vi "NPC3SG Labview V8.5.vi"(0 "dc level 1 in":refnum<vi>, 1 "dc level 2 in":refnum<vi>, 2 "dc level 3 in":refnum<vi>, 3 "loop 1 in":refnum<vi>, 4 "loop 2 in":refnum<vi>, 5 "loop 3 in":refnum<vi>, 6 "Port":refnum<visa-resource-name>="COM1", 7 "command in":refnum<vi>, 14 "dc level 1 out":refnum<vi>, 15 "dc level 2 out":refnum<vi>, 16 "dc level 3 out":refnum<vi>) -> ()   [LabVIEW 2015]
uses:
  SubNPC3SG.llb/device variables.vi
panel:
  in  "Stopp":bool
  in  "Registerkarte":T1(tab)
  in  "Loop 2":bool caption="Loop"
  in  "Remote 2":bool caption="Remote"
  in  "Loop 1":bool caption="Loop"
  in  "Remote 1":bool caption="Remote"
  in  "Remote 0":bool caption="Remote"
  in  "Loop 0":bool caption="Loop"
  in  "Refresh":bool
  out "Serial Number":string="RS232"
  out "Firmware Release Date":string="RS232"
  out "Version Number":string="RS232"
  out "Device":string="RS232"
  in  "com-write":bool caption="Logging"
  out "Receive Buffer":string
  out "Send Buffer":string
  in  "SendString":string caption="Enter Command"
  in  "Send":bool caption="Temp"
  in  "Clear":bool caption="Temp"
  out "Last Error":string="RS232"
  out "Last Command":string="RS232" caption="Command"
  in  "save sequence":bool caption="Loop"
  in  "load sequence":bool caption="Loop"
  in  "start sequence":bool caption="Loop"
  in  "sequence string":string
  in  "Drehschalter 2":dbl(knob) caption="2" min=-10.0 max=90.0 scale=0.0..100.0 scale format="%.3f"
  in  "Drehschalter 1":dbl(knob) caption="1" min=-10.0 max=90.0 scale=0.0..100.0 scale format="%.3f"
  in  "Drehschalter 0":dbl(knob) caption="0" min=-10.0 max=90.0 scale=0.0..100.0 scale format="%.3f"
  # "Piezo 1"
  # "Piezo 2"
  # "Piezo 3"
  # "Loop"
  # "Remote"
  # "possible commands in sequence\n\nset,1,2.34 (actuator position)\nwait,5  - (holding time in sec.)\nstop - (terminate sequence)\n\nexample:\nset,1,2.134\nwait,5\nset,0,22.66\nwait,10\nstop"
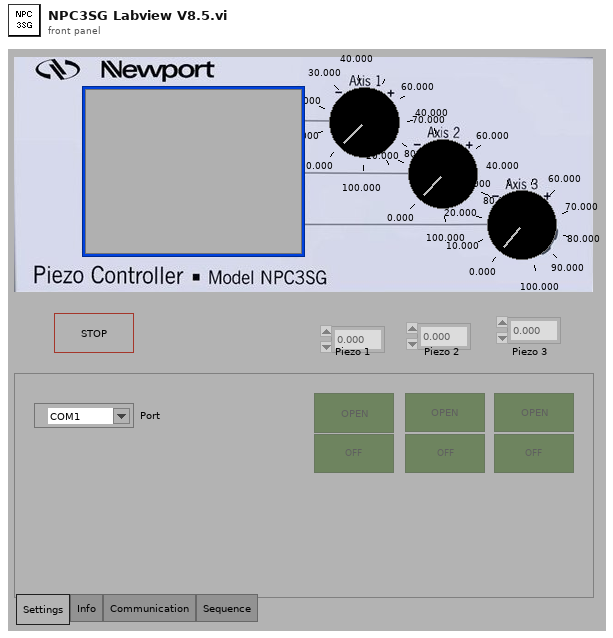
[diagram p1: front panel]
types:
  T1 = enum32{"Settings", "Info", "Communication", "Sequence"}
  T2 = enum16{"open", "replace", "create", "open or create", "replace or create", "replace or create with confirmation"}
  T3 = cluster{"Registerkarte":refnum<vi>, "Array IsActor":bool[], "Array loop":bool[], "Array remote":bool[]}
  T4 = cluster{"Array dc-level":dbl[], "VAR Temp":string, "VAR USB":string, "Array IsActor":bool[], "Array actor-name":string[], "Array axis":string[], "Array loop":bool[], "Array remote":bool[], "Array ovl":bool[]}
  T5 = cluster{"Drehschalter 0":refnum<vi>, "Drehschalter 1":refnum<vi>, "Drehschalter 2":refnum<vi>, "Array loop":bool[], "Array IsActor":bool[], "Array clmin":dbl[], "Array clmax":dbl[], "VAR Vmin":dbl, "VAR Vmax":dbl, "Array dc-level open":dbl[], "Array dc-level closed":dbl[], "VAR actualisation":bool}
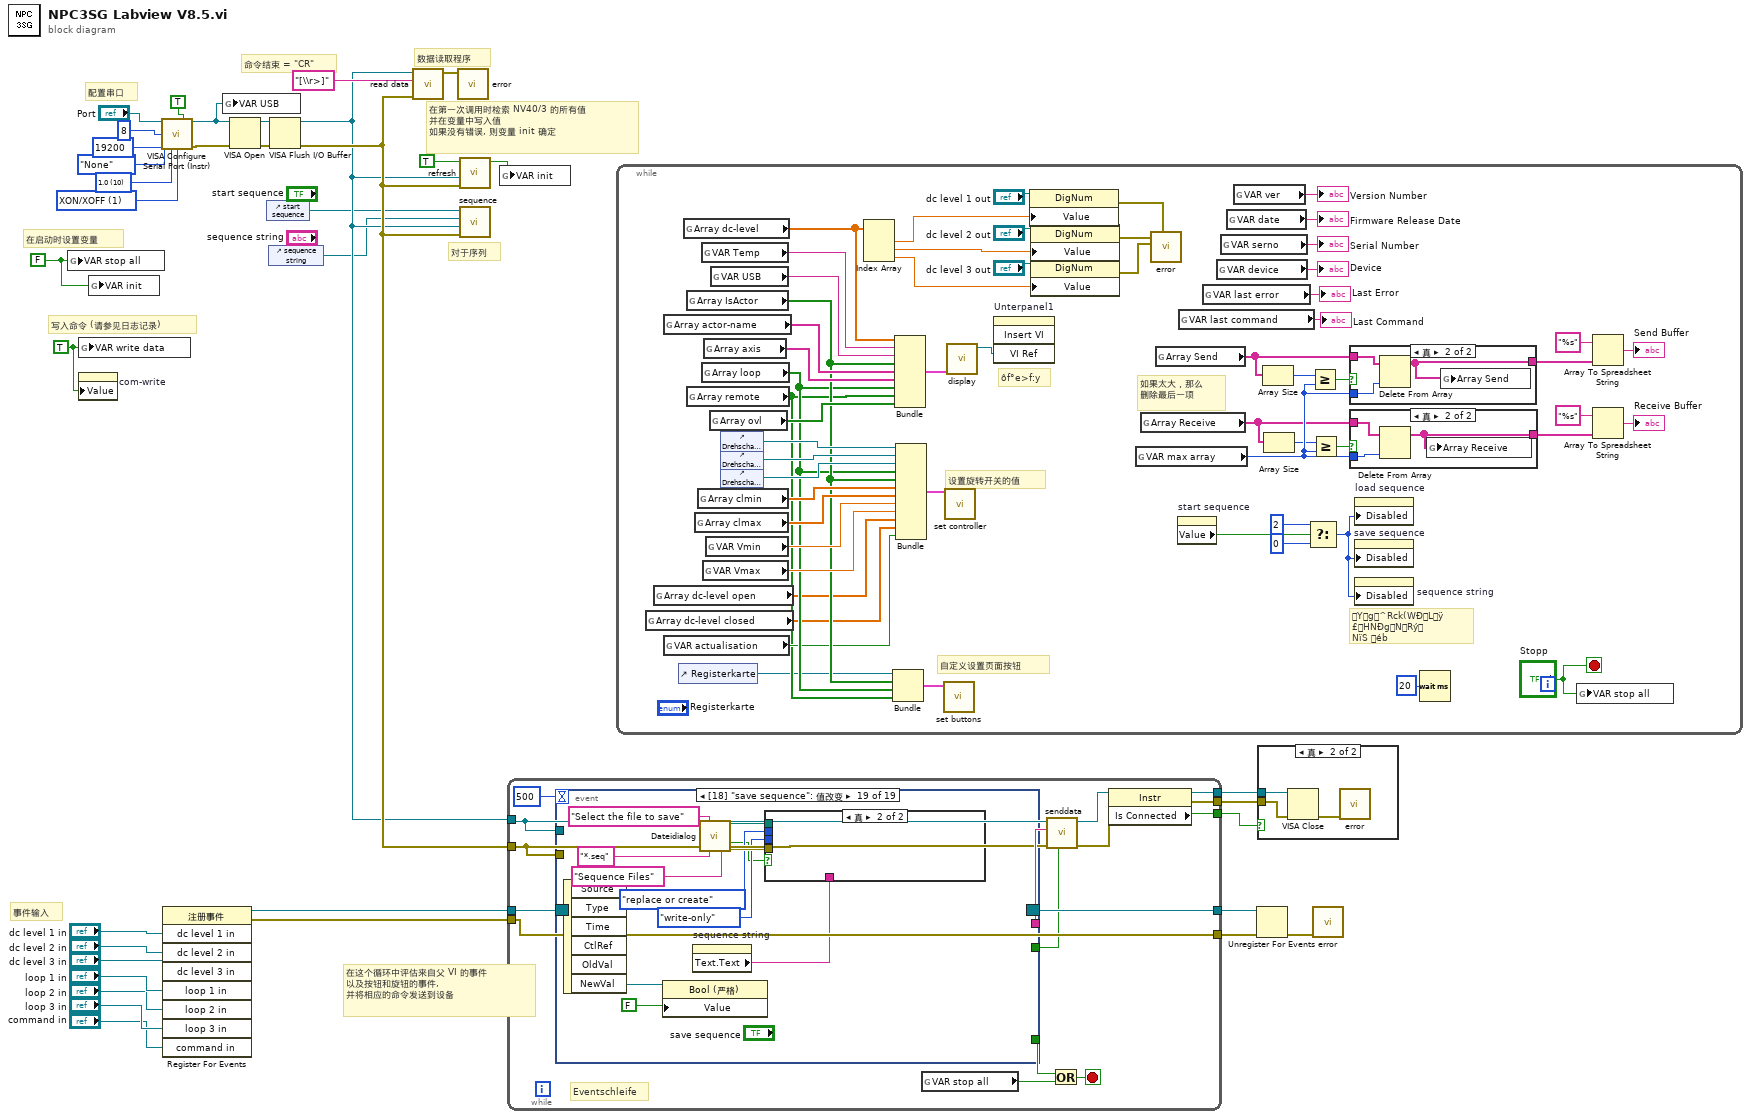
[diagram p0: block diagram]
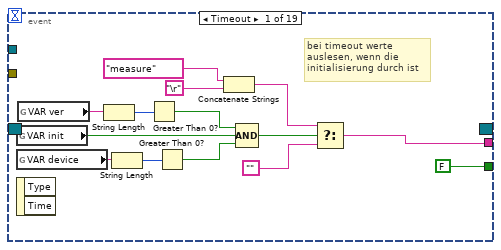
[diagram p3: hidden frame]
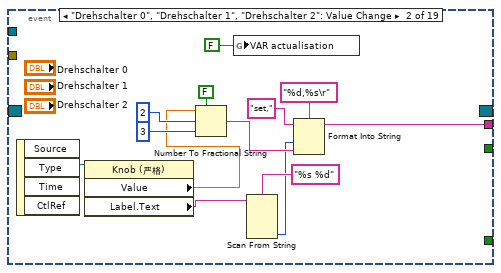
[diagram p4: hidden frame]
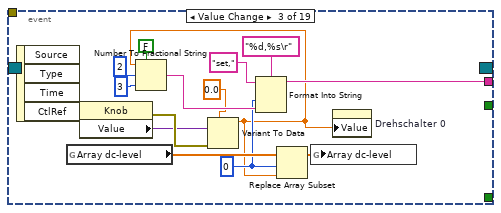
[diagram p5: hidden frame]
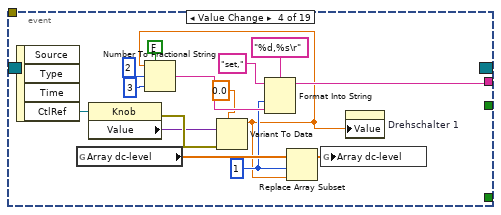
[diagram p6: hidden frame]
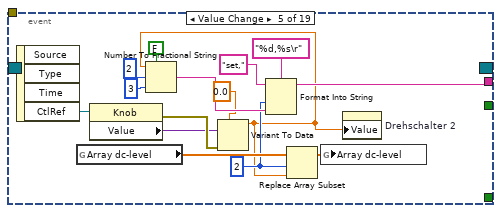
[diagram p7: hidden frame]
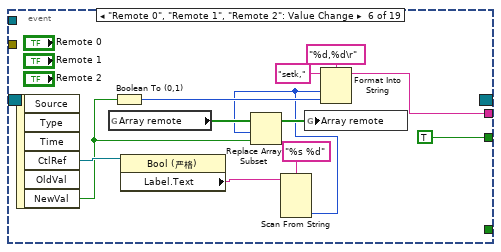
[diagram p8: hidden frame]
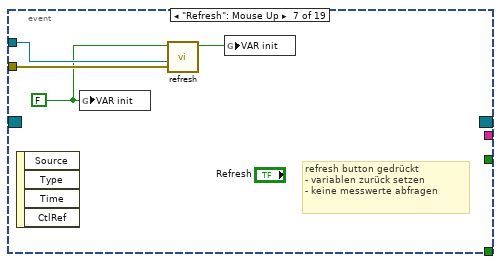
[diagram p9: hidden frame]
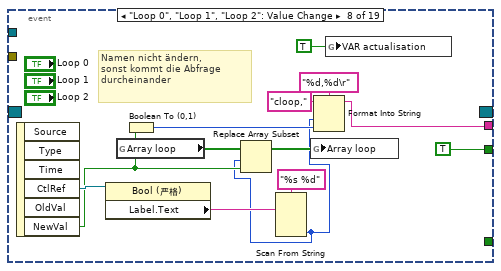
[diagram p10: hidden frame]
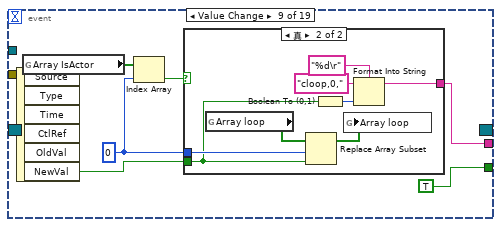
[diagram p11: hidden frame]
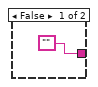
[diagram p12: hidden frame]
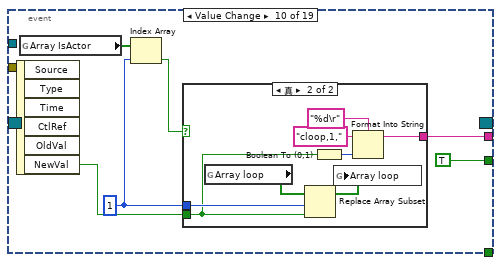
[diagram p13: hidden frame]
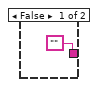
[diagram p14: hidden frame]
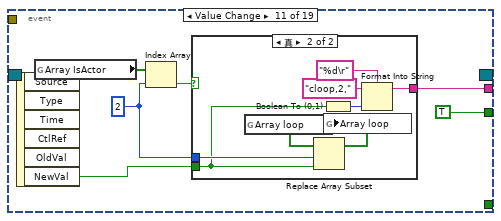
[diagram p15: hidden frame]
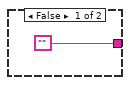
[diagram p16: hidden frame]
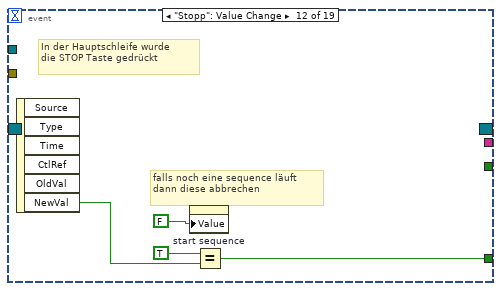
[diagram p17: hidden frame]
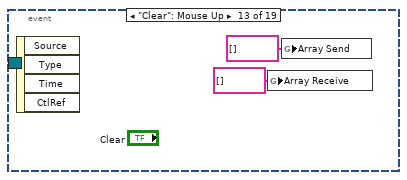
[diagram p18: hidden frame]
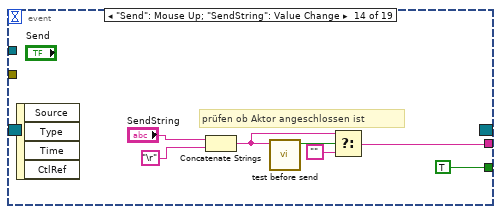
[diagram p19: hidden frame]
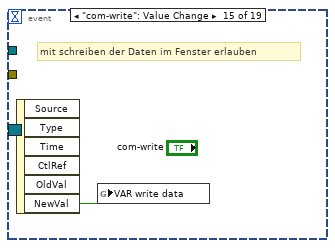
[diagram p20: hidden frame]
diagram:
  w9 = TRUE ("VAR write data")
  w13 = FALSE ("VAR ovl 3")
  w10 = u16 1 items=["Kein", "XON/XOFF", "RTS/CTS", "XON/XOFF & RTS/CTS", "DTR/DSR", "XON/XOFF & DTR/DSR"] ("flow control (0:none)")
  w29 = u16 10 items=["1.0"=10, "1.5"=15, "2.0"=20] ("stop bits (10: 1 bit)")
  # "对于序列"
  # "写入命令 (请参见日志记录)"
  # "命令结束 = \"CR\""
  # "数据读取程序"
  # "在第一次调用时检索 NV40/3 的所有值\n并在变量中写入值\n如果没有错误, 则变量 init 确定"
  # "在启动时设置变量"
  # "配置串口"
  # "事件输入"
  # "在这个循环中评估来自父 VI 的事件\n以及按钮和旋钮的事件, \n并将相应的命令发送到设备"
  n1 = global write "device variables.vi" "VAR stop all"(w13) -> ()
  n2 = global write "device variables.vi" "VAR write data"(w9) -> ()
  n3 = property on="com-write" class="Bool (严格)"("Value"=w9) -> ()  [unwired: 2 in, 2 out]
  n4 = global write "device variables.vi" "VAR init"(w13) -> ()
  n5 = call <vilib>:"VISA Configure Serial Port (Instr).vi"("VISA resource name"="Port", "Enable Termination\nChar (T)"=TRUE ("Enable Termination\nChar (T)"), "baud rate (9600)"=u32 19200, "data bits (8)"=u16 8, "parity (0:none)"=enum16{"None", "Odd", "Even", "Mark", "Space"}."None", "stop bits (10: 1 bit)"=w29, "flow control (0:none)"=w10) -> ("VISA resource name out"=w6:refnum<visa-resource-name>, "error out"=w18:errorcluster)  [unwired: 7 in]
  n6 = register-events("dc level 1 in", "dc level 2 in", "dc level 3 in", "loop 1 in", "loop 2 in", "loop 3 in", "command in") -> (reference out=w35:refnum<event-registration>, error out=w24:errorcluster)  [unwired: 2 in]
  n7 = global write "device variables.vi" "VAR USB"(w6) -> ()
  n8 = VISA Open(error in (no error)=w18, VISA resource name=w6) -> (VISA resource name=w19:refnum<visa-resource-name>, error out=w20:errorcluster)  [unwired: 3 in]
  n9 = control-ref of="start sequence"() -> (w2:refnum<vi>)
  n10 = control-ref of="sequence string"() -> (w1:refnum<vi>)
  n11 = VISA Flush I/O Buffer(VISA resource name=w19, error in (no error)=w20) -> (VISA resource name out=w3:refnum<visa-resource-name>, error out=w4:errorcluster)  [unwired: 1 in]
  n12 = call "read data.vi"("VISA resource name in"=w3, "String End"="[\\r>]", "error in"=w4) -> ("error ende"=w11:errorcluster)  [unwired: 7 in]
  n13 = call "error.vi"("error 1"=w11) -> ()  [unwired: 11 in]
  n14 = call "refresh.vi"("error in"=w4, "VISA-Ressourcen-Name (In)"=w3, "reset all"=TRUE) -> ("init ok??"=w8:bool)  [unwired: 8 in]
  n15 = call "sequence.vi"("error in"=w4, "VISA-Ressourcen-Name"=w3, "Kommandozeilen Refnum"=w1, "Startbutton Refnum"=w2) -> ()  [unwired: 8 in]
  n16 = global write "device variables.vi" "VAR init"(w8) -> ()
  n17 = while {
    tunnel: w4 -> [w38]
    tunnel: w3 -> [w39]
    tunnel: w35 -> [w47]
    tunnel: w24 -> [w40]
    tunnel: [w46] -> w23
    tunnel: [w40] -> w22
    tunnel: [w43] -> w16
    tunnel: [w42] -> w15
    tunnel: [w41] -> w14
    stop <- w49 stop-if-true
    # "Eventschleife"
    n18 = event shown="[18] \"save sequence\": 值改变" {
      selector: w47 -> [_ _ _ _ _ _ _ _ _ _ _ _ _ _ _ _ _ _ _]
      dyn-events: [_ _ _ _ _ _ _ _ _ _ _ _ _ _ _ _ _ _ _] -> w46
      timeout: 500 -> [_ _ _ _ _ _ _ _ _ _ _ _ _ _ _ _ _ _ _]
      tunnel: [w58 w74 w87 w99 w114 w129 _ w141 w157 w174 w188 _ _ w207 _ w214 _ _ _] -> w52
      tunnel: [_ _ _ _ _ _ _ _ _ _ _ w201 _ _ _ _ _ _ _] -> w51
      tunnel: w39 -> [_ _ _ _ _ _ w140 _ _ _ _ _ _ _ _ _ _ _ _]
      tunnel: w38 -> [_ _ _ _ _ _ w139 _ _ _ _ _ _ _ _ _ _ _ _]
      tunnel: [FALSE _ _ _ _ TRUE _ TRUE TRUE TRUE TRUE _ _ TRUE _ TRUE _ _ _] -> w37
      event Timeout {
        # "bei timeout werte auslesen, wenn die initialisierung durch ist"
        n19 = global read "device variables.vi" "VAR init"() -> (w64:bool)
        n20 = global read "device variables.vi" "VAR device"() -> (w62:string)
        n21 = event-data() -> ()  [unwired: 1 in, 2 out]
        n22 = global read "device variables.vi" "VAR ver"() -> (w66:string)
        n23 = String Length(string=w66) -> (length=w65:i32)
        n24 = String Length(string=w62) -> (length=w63:i32)
        n25 = Greater Than 0?(x=w65) -> (x > 0?=w60:bool)
        n26 = Greater Than 0?(x=w63) -> (x > 0?=w61:bool)
        n27 = Concatenate Strings("measure" ("String"), "\r") -> (w55:string)
        n28 = Compound Arithmetic op=AND(w60, w64, w61) -> (w59:bool)
        n29 = Select(t=w55, s=w59, f="") -> (s? t:f=w58:string)
      }
      event "Drehschalter 0", "Drehschalter 1", "Drehschalter 2": Value Change {
        n30 = event-data() -> ("CtlRef"=w73:refnum<vi>)  [unwired: 1 in, 3 out]
        n31 = property class="Knob (严格)"(reference=w73) -> ("Value"=w69:dbl, "Label.Text"=w72:string)  [unwired: 1 in, 2 out]
        n32 = Number To Fractional String(use system decimal point (T)=FALSE ("Systemdezimalzeichen verwenden (T)"), number=w69, width (-)=i16 2 ("Breite (-)"), precision (6)=i16 3 ("Genauigkeit (6)")) -> (F-format string=w70:string)
        n33 = global write "device variables.vi" "VAR actualisation"(FALSE ("VAR mode changed")) -> ()
        n34 = Scan From String(format string="%s %d" ("Format-String"), input string=w72) -> (output 2=w68:i32)  [unwired: 5 in, 3 out]
        n35 = Format Into String(format string="%d,%s\r", initial string="set,", w68, w70) -> (resulting string=w74:string)  [unwired: 1 in, 1 out]
      }
      event Value Change {
        w81 = u8 0 ("Eingang 1")
        n36 = event-data() -> ("CtlRef"=w94:refnum<vi>)  [unwired: 1 in, 3 out]
        n37 = global read "device variables.vi" "Array dc-level"() -> (w83:dbl[])
        n38 = property class="Knob"(reference=w94) -> (error out=w86:errorcluster, "Value"=w85:variant)  [unwired: 1 in, 1 out]
        n39 = Variant To Data(error in=w86, type=0.0, Variant=w85) -> (data=w80:dbl)  [unwired: 1 out]
        n40 = Number To Fractional String(use system decimal point (T)=FALSE ("Systemdezimalzeichen verwenden (T)"), number=w80, width (-)=i16 2 ("Breite (-)"), precision (6)=i16 3 ("Genauigkeit (6)")) -> (F-format string=w88:string)
        n41 = Format Into String(format string="%d,%s\r", initial string="set,", w81, w88) -> (resulting string=w87:string)  [unwired: 1 in, 1 out]
        n42 = Replace Array Subset(array=w83, new element=w80, index=w81) -> (w82:dbl[])
        n43 = global write "device variables.vi" "Array dc-level"(w82) -> ()
        n44 = property on="Drehschalter 0" class="Knob (严格)"("Value"=w80) -> ()  [unwired: 2 in, 2 out]
      }
      event Value Change {
        w96 = u8 1 ("Eingang 1")
        n45 = event-data() -> ("CtlRef"=w100:refnum<vi>)  [unwired: 1 in, 3 out]
        n46 = global read "device variables.vi" "Array dc-level"() -> (w98:dbl[])
        n47 = property class="Knob"(reference=w100) -> (error out=w103:errorcluster, "Value"=w102:variant)  [unwired: 1 in, 1 out]
        n48 = Variant To Data(error in=w103, type=0.0, Variant=w102) -> (data=w95:dbl)  [unwired: 1 out]
        n49 = Number To Fractional String(use system decimal point (T)=FALSE ("Systemdezimalzeichen verwenden (T)"), number=w95, width (-)=i16 2 ("Breite (-)"), precision (6)=i16 3 ("Genauigkeit (6)")) -> (F-format string=w104:string)
        n50 = Format Into String(format string="%d,%s\r", initial string="set,", w96, w104) -> (resulting string=w99:string)  [unwired: 1 in, 1 out]
        n51 = Replace Array Subset(array=w98, new element=w95, index=w96) -> (w97:dbl[])
        n52 = global write "device variables.vi" "Array dc-level"(w97) -> ()
        n53 = property on="Drehschalter 1" class="Knob (严格)"("Value"=w95) -> ()  [unwired: 2 in, 2 out]
      }
      event Value Change {
        w111 = u8 2 ("Eingang 1")
        n54 = event-data() -> ("CtlRef"=w115:refnum<vi>)  [unwired: 1 in, 3 out]
        n55 = global read "device variables.vi" "Array dc-level"() -> (w113:dbl[])
        n56 = property class="Knob"(reference=w115) -> (error out=w118:errorcluster, "Value"=w117:variant)  [unwired: 1 in, 1 out]
        n57 = Variant To Data(error in=w118, type=0.0, Variant=w117) -> (data=w110:dbl)  [unwired: 1 out]
        n58 = Number To Fractional String(use system decimal point (T)=FALSE ("Systemdezimalzeichen verwenden (T)"), number=w110, width (-)=i16 2 ("Breite (-)"), precision (6)=i16 3 ("Genauigkeit (6)")) -> (F-format string=w119:string)
        n59 = Format Into String(format string="%d,%s\r", initial string="set,", w111, w119) -> (resulting string=w114:string)  [unwired: 1 in, 1 out]
        n60 = Replace Array Subset(array=w113, new element=w110, index=w111) -> (w112:dbl[])
        n61 = global write "device variables.vi" "Array dc-level"(w112) -> ()
        n62 = property on="Drehschalter 2" class="Knob (严格)"("Value"=w110) -> ()  [unwired: 2 in, 2 out]
      }
      event "Remote 0", "Remote 1", "Remote 2": Value Change {
        n63 = event-data() -> ("CtlRef"=w134:refnum<vi>, "NewVal"=w126:bool)  [unwired: 1 in, 4 out]
        n64 = global read "device variables.vi" "Array remote"() -> (w135:bool[])
        n65 = Boolean To (0,1)(Boolean=w126) -> (0, 1=w130:i16)
        n66 = property class="Bool (严格)"(reference=w134) -> ("Label.Text"=w127:string)  [unwired: 1 in, 2 out]
        n67 = Scan From String(format string="%s %d" ("Format-String"), input string=w127) -> (output 2=w128:i32)  [unwired: 5 in, 3 out]
        n68 = Replace Array Subset(array=w135, new element=w126, index=w128) -> (w136:bool[])
        n69 = global write "device variables.vi" "Array remote"(w136) -> ()
        n70 = Format Into String(format string="%d,%d\r" ("Format-String"), initial string="setk,", w128, w130) -> (resulting string=w129:string)  [unwired: 1 in, 1 out]
      }
      event "Refresh": Mouse Up {
        w138 = FALSE ("VAR init")
        # "refresh button gedrückt\n- variablen zurück setzen\n- keine messwerte abfragen"
        n71 = event-data() -> ()  [unwired: 1 in, 4 out]
        n72 = global write "device variables.vi" "VAR init"(w138) -> ()
        n73 = call "refresh.vi"("error in"=w139, "VISA-Ressourcen-Name (In)"=w140, "reset all"=w138) -> ("init ok??"=w137:bool)  [unwired: 8 in]
        n74 = global write "device variables.vi" "VAR init"(w137) -> ()
      }
      event "Loop 0", "Loop 1", "Loop 2": Value Change {
        # "Namen nicht ändern,\nsonst kommt die Abfrage\ndurcheinander"
        n75 = event-data() -> ("CtlRef"=w147:refnum<vi>, "NewVal"=w146:bool)  [unwired: 1 in, 4 out]
        n76 = property class="Bool (严格)"(reference=w147) -> ("Label.Text"=w145:string)  [unwired: 1 in, 2 out]
        n77 = global read "device variables.vi" "Array loop"() -> (w152:bool[])
        n78 = Boolean To (0,1)(Boolean=w146) -> (0, 1=w148:i16)
        n79 = Scan From String(format string="%s %d" ("Format-String"), input string=w145) -> (output 2=w144:i32)  [unwired: 5 in, 3 out]
        n80 = Replace Array Subset(array=w152, new element=w146, index=w144) -> (w153:bool[])
        n81 = global write "device variables.vi" "Array loop"(w153) -> ()
        n82 = Format Into String(format string="%d,%d\r" ("Format-String"), initial string="cloop,", w144, w148) -> (resulting string=w141:string)  [unwired: 1 in, 1 out]
        n83 = global write "device variables.vi" "VAR actualisation"(TRUE ("VAR mode changed")) -> ()
      }
      event Value Change {
        w155 = 0 ("Index")
        n84 = event-data() -> ("NewVal"=w156:bool)  [unwired: 1 in, 5 out]
        n85 = global read "device variables.vi" "Array IsActor"() -> (w159:bool[])
        n86 = Index Array(array=w159, index=w155) -> (element=w158:bool)
        n87 = case shown="真" w158 {
          tunnel: ["" w166] -> w157
          tunnel: w156 -> [_ w161]
          tunnel: w155 -> [_ w163]
          frame False {
          }
          frame True {
            n88 = global read "device variables.vi" "Array loop"() -> (w165:bool[])
            n89 = Replace Array Subset(array=w165, new element=w161, index=w163) -> (w164:bool[])
            n90 = Boolean To (0,1)(Boolean=w161) -> (0, 1=w162:i16)
            n91 = global write "device variables.vi" "Array loop"(w164) -> ()
            n92 = Format Into String(format string="%d\r" ("Format-String"), initial string="cloop,0," ("Anfangsstring"), w162) -> (resulting string=w166:string)  [unwired: 1 in, 1 out]
          }
        }
      }
      event Value Change {
        w170 = 1
        n93 = event-data() -> ("NewVal"=w171:bool)  [unwired: 1 in, 5 out]
        n94 = global read "device variables.vi" "Array IsActor"() -> (w173:bool[])
        n95 = Index Array(array=w173, index=w170) -> (element=w172:bool)
        n96 = case shown="真" w172 {
          tunnel: ["" w181] -> w174
          tunnel: w171 -> [_ w176]
          tunnel: w170 -> [_ w178]
          frame False {
          }
          frame True {
            n97 = global read "device variables.vi" "Array loop"() -> (w180:bool[])
            n98 = Replace Array Subset(array=w180, new element=w176, index=w178) -> (w179:bool[])
            n99 = Boolean To (0,1)(Boolean=w176) -> (0, 1=w177:i16)
            n100 = global write "device variables.vi" "Array loop"(w179) -> ()
            n101 = Format Into String(format string="%d\r" ("Format-String"), initial string="cloop,1," ("Anfangsstring"), w177) -> (resulting string=w181:string)  [unwired: 1 in, 1 out]
          }
        }
      }
      event Value Change {
        w185 = 2
        n102 = event-data() -> ("NewVal"=w186:bool)  [unwired: 1 in, 5 out]
        n103 = global read "device variables.vi" "Array IsActor"() -> (w189:bool[])
        n104 = Index Array(array=w189, index=w185) -> (element=w187:bool)
        n105 = case shown="真" w187 {
          tunnel: ["" w196] -> w188
          tunnel: w186 -> [_ w191]
          tunnel: w185 -> [_ w193]
          frame False {
          }
          frame True {
            n106 = global read "device variables.vi" "Array loop"() -> (w195:bool[])
            n107 = Replace Array Subset(array=w195, new element=w191, index=w193) -> (w194:bool[])
            n108 = Boolean To (0,1)(Boolean=w191) -> (0, 1=w192:i16)
            n109 = global write "device variables.vi" "Array loop"(w194) -> ()
            n110 = Format Into String(format string="%d\r" ("Format-String"), initial string="cloop,2," ("Anfangsstring"), w192) -> (resulting string=w196:string)  [unwired: 1 in, 1 out]
          }
        }
      }
      event "Stopp": Value Change {
        # "falls noch eine sequence läuft\ndann diese abbrechen"
        # "In der Hauptschleife wurde\ndie STOP Taste gedrückt"
        n111 = event-data() -> ("NewVal"=w202:bool)  [unwired: 1 in, 5 out]
        n112 = property on="start sequence" class="Bool (严格)"("Value"=FALSE ("start sequence")) -> ()  [unwired: 2 in, 2 out]
        n113 = Equal?(x=TRUE, y=w202) -> (x = y?=w201:bool)
      }
      event "Clear": Mouse Up {
        n114 = event-data() -> ()  [unwired: 1 in, 4 out]
        n115 = global write "device variables.vi" "Array Receive"(string[] [] ("Array Receive")) -> ()
        n116 = global write "device variables.vi" "Array Send"(string[] [] ("Array Send")) -> ()
      }
      event "Send": Mouse Up; "SendString": Value Change {
        # "prüfen ob Aktor angeschlossen ist"
        n117 = event-data() -> ()  [unwired: 1 in, 4 out]
        n118 = Concatenate Strings("SendString", "\r") -> (w208:string)
        n119 = call "test before send.vi"("data string in"=w208) -> ("send OK"=w209:bool)  [unwired: 10 in]
        n120 = Select(t=w208, s=w209, f="") -> (s? t:f=w207:string)
      }
      event "com-write": Value Change {
        # "mit schreiben der Daten im Fenster erlauben"
        n121 = event-data() -> ("NewVal"=w212:bool)  [unwired: 1 in, 5 out]
        n122 = global write "device variables.vi" "VAR write data"(w212) -> ()
      }
      event Value Change {
        # "prüfen, ob Aktor angeschlossen"
        # "Kommando wurde von aussen geschickt"
        n123 = event-data() -> ("NewVal"=w219:string)  [unwired: 1 in, 5 out]
        n124 = Concatenate Strings(w219, "\r") -> (w216:string)
        n125 = call "test before send.vi"("data string in"=w216) -> ("send OK"=w217:bool)  [unwired: 10 in]
        n126 = Select(t=w216, s=w217, f="") -> (s? t:f=w214:string)
      }
      event "start sequence": Value Change {
        n127 = event-data() -> ()  [unwired: 1 in, 6 out]
      }
      event "load sequence": Value Change {
        n128 = event-data() -> ("CtlRef"=w221:refnum<vi>)  [unwired: 1 in, 5 out]
        n129 = property class="Bool (严格)"(reference=w221, "Value"=FALSE ("Wert")) -> ()  [unwired: 1 in, 2 out]
        n130 = call "Dateidialog2"("prompt"="Select the file to load", "pattern (all files)"="*.seq", "pattern label"="Sequence Files") -> ("selected path"=w227:path, "exists"=w223:bool, "error out"=w226:errorcluster)  [unwired: 9 in, 1 out]
        n131 = case shown="真" w223 {
          tunnel: w227 -> [_ w241]
          tunnel: w226 -> [_ w240]
          tunnel: T2."open" ("Operation (0:Öffnen)") -> [_ w238]
          tunnel: enum16{"read/write", "read-only", "write-only"}."read-only" ("Zugriff (0:Lesen/Schreiben)") -> [_ w237]
          tunnel: [w231 w232] -> w222
          frame False {
            (unwired) ""
            n132 = property on="sequence string" class="Str"() -> ("Text.Text"=w231:string)  [unwired: 2 in, 2 out]
          }
          frame True {
            n133 = Open/Create/Replace File(file path (use dialog)=w241, error in=w240, operation (0:open)=w238, access (0:read/write)=w237) -> (refnum out=w234:refnum<file>, error out=w233:errorcluster)  [unwired: 2 in, 1 out]
            n134 = Read from Text File(file (use dialog)=w234, error in=w233) -> (refnum out=w235:refnum<file>, text=w232:string, error out=w236:errorcluster)  [unwired: 2 in, 1 out]
            n135 = Close File(refnum=w235, error in=w236) -> (error out=w239:errorcluster)  [unwired: 1 out]
            n136 = call <vilib>:"Simple Error Handler.vi"("error in (no error)"=w239) -> ()  [unwired: 4 in, 5 out]
          }
        }
        n137 = property on="sequence string" class="Str"("Text.Text"=w222) -> ()  [unwired: 2 in, 2 out]
      }
      event "save sequence": Value Change {
        n138 = event-data() -> ("CtlRef"=w244:refnum<vi>)  [unwired: 1 in, 5 out]
        n139 = property class="Bool (严格)"(reference=w244, "Value"=FALSE ("Wert")) -> ()  [unwired: 1 in, 2 out]
        n140 = property on="sequence string" class="Str"() -> ("Text.Text"=w247:string)  [unwired: 2 in, 2 out]
        n141 = call "Dateidialog"("prompt"="Select the file to save", "pattern (all files)"="*.seq", "pattern label"="Sequence Files") -> ("selected path"=w249:path, "cancelled"=w242:bool, "error out"=w248:errorcluster)  [unwired: 9 in, 1 out]
        n142 = case shown="真" w242 {
          tunnel: w249 -> [w262 _]
          tunnel: w248 -> [w261 _]
          tunnel: w247 -> [w260 _]
          tunnel: T2."replace or create" ("Operation (0:Öffnen)") -> [w259 _]
          tunnel: enum16{"read/write", "read-only", "write-only"}."write-only" ("Zugriff (0:Lesen/Schreiben)") -> [w258 _]
          frame False {
            n143 = Open/Create/Replace File(file path (use dialog)=w262, error in=w261, operation (0:open)=w259, access (0:read/write)=w258) -> (refnum out=w257:refnum<file>, error out=w254:errorcluster)  [unwired: 2 in, 1 out]
            n144 = Write to Text File(file (use dialog)=w257, text=w260, error in=w254) -> (refnum out=w255:refnum<file>, error out=w256:errorcluster)  [unwired: 1 in, 1 out]
            n145 = Close File(refnum=w255, error in=w256) -> (error out=w253:errorcluster)  [unwired: 1 out]
            n146 = call <vilib>:"Simple Error Handler.vi"("error in (no error)"=w253) -> ()  [unwired: 4 in, 5 out]
          }
          frame True {
          }
        }
      }
    }
    n147 = global read "device variables.vi" "VAR stop all"() -> (w50:bool)
    n148 = call "senddata.vi"("read ERR"=w37, "error in"=w38, "writebuffer"=w52, "VISA-Ressourcen-Name"=w39) -> ("error out"=w44:errorcluster, "VISA-Ressourcen-Name (Ausgang)"=w45:refnum<visa-resource-name>)  [unwired: 5 in, 1 out]
    n149 = Or(x=w51, y=w50) -> (x .or. y?=w49:bool)
    n150 = property class="Instr"(reference=w45, error in=w44) -> (reference out=w43:refnum<visa-resource-name>, error out=w42:errorcluster, "Is Connected"=w41:bool)
  }
  n151 = while {
    stop <- "Stopp" stop-if-true
    # "Yg^Rck(WÐLÿ\n£HNÐgNRý\nNïS\téb"
    # "如果太大，那么\n删除最后一项"
    # "ôf°e>f:y"
    # "自定义设置页面按钮"
    # "设置旋转开关的值"
    n152 = global read "device variables.vi" "Array dc-level closed"() -> (w274:dbl[])
    n153 = global read "device variables.vi" "Array dc-level open"() -> (w275:dbl[])
    n154 = global read "device variables.vi" "Array actor-name"() -> (w316:string[])
    n155 = global read "device variables.vi" "VAR actualisation"() -> (w272:bool)
    n156 = control-ref of="Registerkarte"() -> (w270:refnum<vi>)
    n157 = global read "device variables.vi" "Array dc-level"() -> (w313:dbl[])
    n158 = global read "device variables.vi" "Array IsActor"() -> (w294:bool[])
    n159 = global read "device variables.vi" "Array remote"() -> (w271:bool[])
    n160 = global read "device variables.vi" "Array clmax"() -> (w301:dbl[])
    n161 = global read "device variables.vi" "Array clmin"() -> (w302:dbl[])
    n162 = global read "device variables.vi" "VAR Temp"() -> (w318:string)
    n163 = global read "device variables.vi" "Array loop"() -> (w293:bool[])
    n164 = global read "device variables.vi" "VAR Vmax"() -> (w299:dbl)
    n165 = global read "device variables.vi" "Array axis"() -> (w315:string[])
    n166 = global read "device variables.vi" "VAR Vmin"() -> (w300:dbl)
    n167 = global read "device variables.vi" "Array ovl"() -> (w314:bool[])
    n168 = global read "device variables.vi" "VAR USB"() -> (w317:string)
    n169 = control-ref of="Drehschalter 0"() -> (w298:refnum<vi>)
    n170 = control-ref of="Drehschalter 1"() -> (w297:refnum<vi>)
    n171 = control-ref of="Drehschalter 2"() -> (w296:refnum<vi>)
    n172 = Index Array(array=w313) -> (element #1=w312:dbl, element #2=w311:dbl, element #3=w310:dbl)  [unwired: 3 in]
    n173 = Bundle("Registerkarte"=w270, "Array IsActor"=w294, "Array loop"=w293, "Array remote"=w271) -> (w269:T3)  [unwired: 1 in]
    n174 = Bundle("Array dc-level"=w313, "VAR Temp"=w318, "VAR USB"=w317, "Array IsActor"=w294, "Array actor-name"=w316, "Array axis"=w315, "Array loop"=w293, "Array remote"=w271, "Array ovl"=w314) -> (w295:T4)  [unwired: 1 in]
    n175 = Bundle("Drehschalter 0"=w298, "Drehschalter 1"=w297, "Drehschalter 2"=w296, "Array loop"=w293, "Array IsActor"=w294, "Array clmin"=w302, "Array clmax"=w301, "VAR Vmin"=w300, "VAR Vmax"=w299, "Array dc-level open"=w275, "Array dc-level closed"=w274, "VAR actualisation"=w272) -> (w273:T5)  [unwired: 1 in]
    n176 = call "set buttons.vi"("Cluster Button"=w269) -> ()  [unwired: 11 in]
    n177 = call "set controller.vi"("Cluster Controller"=w273) -> ()  [unwired: 12 in, 3 out]
    n178 = call "display.vi"("Cluster Display In"=w295) -> ("Display - Refnum"=w319:refnum<vi>)  [unwired: 10 in]
    n179 = invoke on="Unterpanel1" class="SubPanel" method="Insert VI"("VI Ref"=w319) -> ()  [unwired: 3 in, 4 out]
    n180 = property class="DigNum"(reference="dc level 1 out", "Value"=w312) -> (error out=w309:errorcluster)  [unwired: 1 in, 1 out]
    n181 = property class="DigNum"(reference="dc level 2 out", "Value"=w311) -> (error out=w308:errorcluster)  [unwired: 1 in, 1 out]
    n182 = property class="DigNum"(reference="dc level 3 out", "Value"=w310) -> (error out=w307:errorcluster)  [unwired: 1 in, 1 out]
    n183 = global read "device variables.vi" "VAR max array"() -> (w284:i32)
    n184 = global read "device variables.vi" "Array Receive"() -> (w283:string[])
    n185 = call "error.vi"("error 5"=w309, "error 2"=w307, "error 1"=w308) -> ()  [unwired: 9 in]
    n186 = global read "device variables.vi" "Array Send"() -> (w282:string[])
    n187 = property on="start sequence" class="Bool (严格)"() -> ("Value"=w266:bool)  [unwired: 2 in, 2 out]
    n188 = global read "device variables.vi" "VAR last command"() -> (→"Last Command":string)
    n189 = global read "device variables.vi" "VAR last error"() -> (→"Last Error":string)
    n190 = global read "device variables.vi" "VAR device"() -> (→"Device":string)
    n191 = global read "device variables.vi" "VAR serno"() -> (→"Serial Number":string)
    n192 = global read "device variables.vi" "VAR date"() -> (→"Firmware Release Date":string)
    n193 = global read "device variables.vi" "VAR ver"() -> (→"Version Number":string)
    n194 = Array Size(array=w282) -> (size(s)=w281:i32)
    n195 = Array Size(array=w283) -> (size(s)=w278:i32)
    n196 = Select(t=u8 2 ("Deaktiviert"), s=w266, f=u8 0) -> (s? t:f=w265:u8)
    n197 = Greater Or Equal?(x=w281, y=w284) -> (x >= y?=w280:bool)
    n198 = Greater Or Equal?(x=w278, y=w284) -> (x >= y?=w279:bool)
    n199 = case shown="真" w280 {
      tunnel: [w321 w322] -> w276
      tunnel: w282 -> [w321 w324]
      tunnel: w284 -> [_ w323]
      frame False {
      }
      frame True {
        n200 = Delete From Array(array=w324, index=w323) -> (array with subset deleted=w322:string[])  [unwired: 1 in, 1 out]
        n201 = global write "device variables.vi" "Array Send"(w322) -> ()
      }
    }
    n202 = case shown="真" w279 {
      tunnel: w284 -> [_ w328]
      tunnel: [w325 w326] -> w277
      tunnel: w283 -> [w325 w327]
      frame False {
      }
      frame True {
        n203 = Delete From Array(array=w327, index=w328) -> (array with subset deleted=w326:string[])  [unwired: 1 in, 1 out]
        n204 = global write "device variables.vi" "Array Receive"(w326) -> ()
      }
    }
    n205 = property on="load sequence" class="Bool (严格)"("Disabled"=w265) -> ()  [unwired: 2 in, 2 out]
    n206 = property on="save sequence" class="Bool (严格)"("Disabled"=w265) -> ()  [unwired: 2 in, 2 out]
    n207 = property on="sequence string" class="Str"("Disabled"=w265) -> ()  [unwired: 2 in, 2 out]
    n208 = Wait (ms)(milliseconds to wait=u32 20 ("Zu wartende ms")) -> ()  [unwired: 1 out]
    n209 = global write "device variables.vi" "VAR stop all"("Stopp") -> ()
    n210 = Array To Spreadsheet String(array=w276, 3:"%s" ("Format-String")) -> (spreadsheet string=→"Send Buffer":string)  [unwired: 1 in]
    n211 = Array To Spreadsheet String(array=w277, 3:"%s" ("Format-String")) -> (spreadsheet string=→"Receive Buffer":string)  [unwired: 1 in]
  }
  n212 = Unregister For Events(event registration refnum=w23, error in=w22) -> (error out=w21:errorcluster)
  n213 = case shown="真" w14 {
    tunnel: w16 -> [_ w331]
    tunnel: w15 -> [_ w330]
    frame False {
    }
    frame True {
      n214 = VISA Close(VISA resource name=w331, error in (no error)=w330) -> (error out=w329:errorcluster)
      n215 = call "error.vi"("error 4"=w329) -> ()  [unwired: 11 in]
    }
  }
  n216 = call "error.vi"("error 4"=w21) -> ()  [unwired: 11 in]
